vi "S2C_5190CR_Poly_MeasurePower.vi"(8 "Error In":errorcluster, 10 "Measure":cluster{"OutletPlug":u16, "Timeout(ms)":i32}={"OutletPlug"=1, "Timeout(ms)"=10000} {"OutletPlug" items=["Outlet 1"=1, "Outlet 2"=2, "Outlet 3"=3, "Outlet 4"=4, "Outlet 5"=5, "Outlet 6"=6, "Outlet 7"=7, "Outlet 8"=8]}, 11 "Settings":T1={"Driver"="5190CR", "Command"="Measure Power", "Return"="Power(W)", "Parameters"="", "Timeout"=10.0}) -> (0 "Error Out":errorcluster, 3 "Response":string)   [LabVIEW 2015]
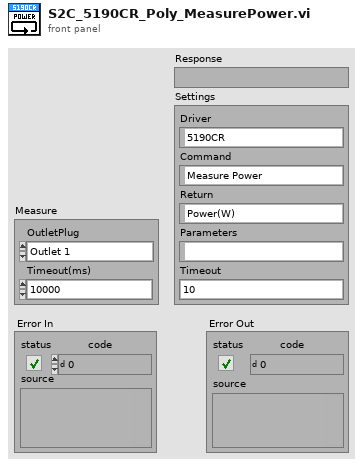
[diagram p1: front panel]
types:
  T1 = cluster{"Driver":string, "Command":string, "Return":string, "Parameters":string, "Timeout":dbl}
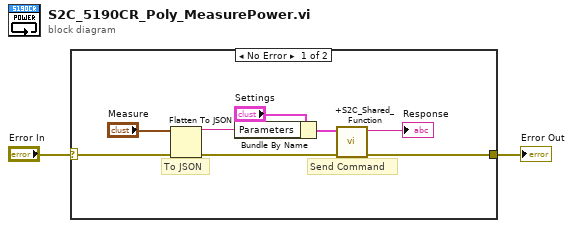
[diagram p0: block diagram]
diagram:
  n1 = case shown="No Error" "Error In" {
    selector: "Error In" -> [w6 w11]
    tunnel: [w5 w11] -> w1
    frame No Error {
      # "To JSON"
      # "Send Command"
      n2 = Flatten To JSON(anything="Measure", error in (no error)=w6) -> (JSON string=w7:string, 11:w9:errorcluster)  [unwired: 1 in]
      n3 = Bundle By Name(cluster="Settings", "Parameters"=w7) -> (w10:T1)
      n4 = call "+S2C_Shared_Function.vi"("Error In"=w9, "Settings"=w10) -> ("Error Out"=w5:errorcluster, "Response"=→"Response":string)  [unwired: 8 in]
    }
    frame Error {
    }
  }
  "Error Out" <- w1
